vi "GV STAGEXasTrigger.vi"() -> ()   [LabVIEW 2017]
panel:
  out "STAGEXasTrig":bool
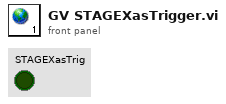
[diagram p1: front panel]
diagram:
